vi "editscenario Export Scenario.vi"(8 "error in (no error)":errorcluster, 10 "sxScenarioId (\"\")":string, 11 "Connection Refnum":T1) -> (0 "error out":errorcluster, 2 "Scenario XML":string, 3 "Connection Refnum":T1)   [LabVIEW 2011]
uses:
  Summitek EXT/ODBC/SQL Controls/Connection Refnum.ctl
  scenario xml.ctl
  server/server lib/Spartan Version.vi
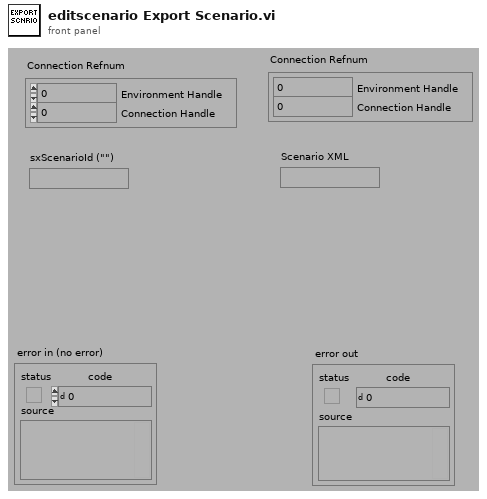
[diagram p1: front panel]
types:
  T1 = typedef "Connection Refnum.ctl" = cluster{"Environment Handle":i32, "Connection Handle":i32}
  T2 = typedef "scenario xml.ctl" = cluster{"#attributes":cluster{"version":string, "creator":string}, "sxScenarioId":string, "sDescription":string, "sLogic":string, "sResultFieldsCSV":string, "sTemplatesCSV":string, "fAutoRunReports":bool, "fSortByTemplates":bool, "fCombinePDF":bool, "Conditions":cluster{"sxFieldId":string, "nOperator":string, "sMatchValue":string}[]}
  T3 = typedef "Scenario Record.ctl" = cluster{"ixScenario":i32, "tCreated":timestamp, "tModified":timestamp, "sxUsername":string, "sModifiedBy":string, "sxScenarioId":string, "sDescription":string, "sLogic":string, "sResultFieldsCSV":string, "sTemplatesCSV":string, "fAutoRunReports":bool, "fSortByTemplates":bool, "fCombinePDF":bool, "Conditions":T4[]}
  T4 = typedef "Condition Record.ctl" = cluster{"iConditionIndex":i32, "sxFieldId":string, "nOperator":T5, "sMatchValue":string}
  T5 = typedef "Condition Operators.ctl" = enum16{"equal (=)", "not equal (\\u2260)", "less than (<)", "less than or equal (\\u2264)", "greater than (>)", "greater than or equal (\\u2265)", "contains", "does not contain"}
  T6 = typedef "OGAB Version.ctl" = cluster{"Version":string, "Build Number":u32, "Build Date/Time":dbl}
  T7 = cluster{"sxFieldId":string, "nOperator":string, "sMatchValue":string}[]
  T8 = cluster{"sxFieldId":string, "nOperator":string, "sMatchValue":string}
  T9 = typedef "Field Record.ctl" = cluster{"ixField":i32, "iSequenceOrder":i32, "sxFieldId":string, "sxSequenceId":string, "sDisplayName":string, "sValue":string, "sUnits":string, "nDataType":T10, "nNextItem":T11, "fSystem":bool, "fSystemValue":bool, "fRequired":bool, "fSetAtTest":bool, "fTestField":bool, "fDeleted":bool, "fIndexed":bool, "fFreeList":bool}
  T10 = typedef "Field DataTypes.ctl" = enum32{"text", "numeric", "list", "timestamp", "boolean"}
  T11 = typedef "Field NextItem.ctl" = enum32{"Reset", "Retain", "Auto-Increment"}
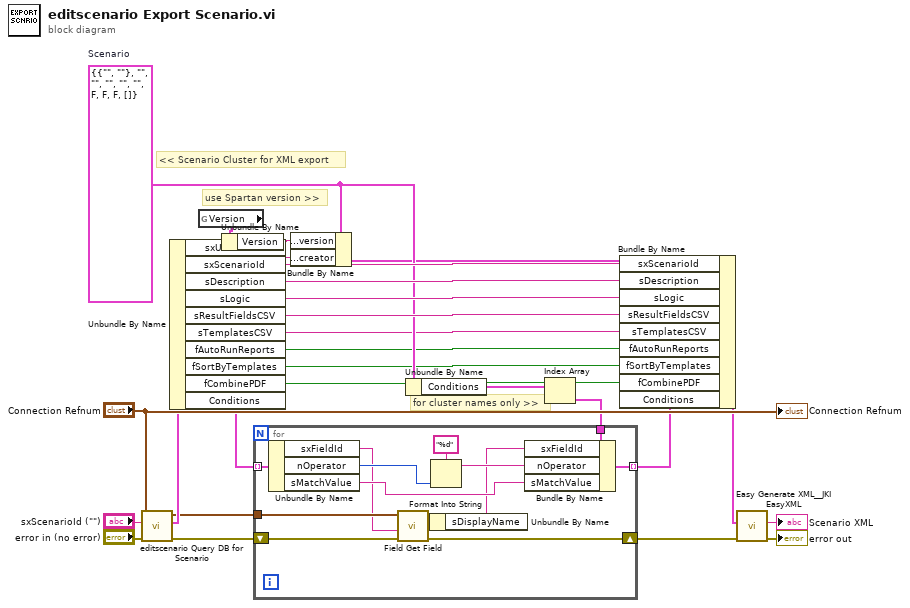
[diagram p0: block diagram]
diagram:
  w14 = T2 {"#attributes"={"version"="", "creator"=""}, "sxScenarioId"="", "sDescription"="", "sLogic"="", "sResultFieldsCSV"="", "sTemplatesCSV"="", "fAutoRunReports"=FALSE, "fSortByTemplates"=FALSE, "fCombinePDF"=FALSE, "Conditions"=[]}  # Scenario
  # "use Spartan version >>"
  # "for cluster names only >>"
  # "<< Scenario Cluster for XML export"
  n1 = call "editscenario Query DB for Scenario.vi"("error in (no error)"="error in (no error)", "sxScenarioId (\"\")"="sxScenarioId (\"\")", "Connection Refnum"="Connection Refnum") -> ("error out"=w7:errorcluster, "Scenario Record"=w24:T3, "Connection Refnum"=w6:T1)  [unwired: 6 out]
  n2 = Unbundle By Name(w24) -> ("sxUsername"=w1:string, "sxScenarioId"=w22:string, "sDescription"=w21:string, "sLogic"=w20:string, "sResultFieldsCSV"=w19:string, "sTemplatesCSV"=w8:string, "fAutoRunReports"=w2:bool, "fSortByTemplates"=w4:bool, "fCombinePDF"=w3:bool, "Conditions"=w18:T4[])
  n3 = global read "Spartan Version.vi" "Version"() -> (w23:T6)
  n4 = Unbundle By Name(w23) -> ("Version"=w12:string)
  n5 = Bundle By Name(cluster=w14, "#attributes.version"=w12, "#attributes.creator"=w1) -> (w13:T2)
  n6 = Unbundle By Name(w14) -> ("Conditions"=w10:T7)
  n7 = Index Array(array=w10) -> (element=w9:T8)  [unwired: 1 in]
  n8 = for {
    tunnel: w18 -> [w40] mode=indexing
    tunnel: w9 -> [w39]
    tunnel: [w38] -> w17 mode=indexing
    shift-right: [w28] -> w5
    shift-left: w7 -> [w32]
    tunnel: w6 -> [w33]
    n9 = Unbundle By Name(w40) -> ("sxFieldId"=w31:string, "nOperator"=w36:T5, "sMatchValue"=w37:string)
    n10 = call "Field Get Field.vi"("error in (no error)"=w32, "sFieldId or sDisplayName (\"\")"=w31, "Connection Refnum"=w33) -> ("error out"=w28:errorcluster, "Field"=w30:T9)  [unwired: 2 in, 5 out]
    n11 = Unbundle By Name(w30) -> ("sDisplayName"=w29:string)
    n12 = Format Into String(format string="%d", w36) -> (resulting string=w34:string)  [unwired: 2 in, 1 out]
    n13 = Bundle By Name(cluster=w39, "sxFieldId"=w29, "nOperator"=w34, "sMatchValue"=w37) -> (w38:T8)
  }
  n14 = Bundle By Name(cluster=w13, "sxScenarioId"=w22, "sDescription"=w21, "sLogic"=w20, "sResultFieldsCSV"=w19, "sTemplatesCSV"=w8, "fAutoRunReports"=w2, "fSortByTemplates"=w4, "fCombinePDF"=w3, "Conditions"=w17) -> (w16:T2)
  n15 = call "Easy Generate XML__JKI EasyXML.vi"("error in (no error)"=w5, "LabVIEW Data"=w16) -> ("error out"=→"error out":errorcluster, "XML String"=→"Scenario XML":string)  [unwired: 8 out]
  "Connection Refnum" <- "Connection Refnum"
